vi "PH_PPMA_PowerUnit.PS Stand by.vi"(0 "i ref in":refnum<vi>, 5 "error in (no error)":errorcluster) -> (14 "i ref out":refnum<vi>, 19 "error out":errorcluster)   [LabVIEW 2014, in "PH_PPMA_PowerUnit.lvlib"]
doc: "This is the entry action of the \"Stand by\" state of the state machine."
uses:
  PH_PPMA_PowerUnit.lvlib
  PH_Devices/PH_Beckhoff_PPMA-Rods/PH_Beckhoff_PPMA-Rods.lvlib
  PH_Devices/PH_Beckhoff_PP_PU/PH_Beckhoff_PP_PU.lvlib
  PH_Basics/PH_PowerUnit_BaseClass/PH_PowerUnit_BaseClass.lvlib
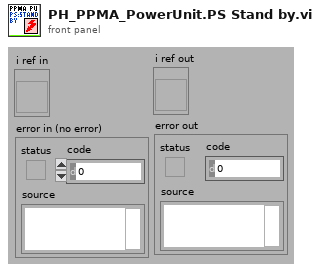
[diagram p1: front panel]
types:
  T1 = typedef "PH_PPMA_PowerUnit.lvlib/PH_PPMA_PowerUnit.i attribute.ctl" = cluster{"GUI Refs":cluster{"Rods":refnum<vi>, "Ignitron":refnum<vi>, "Rossrelais":refnum<vi>, "Set Voltage":refnum<vi>, "PSU":refnum<vi>, "EOC":refnum<vi>, "Trigger":refnum<vi>}, "Rods":T2, "PSU":T4, "Ross Relais":T5, "Ignitron":T6, "Trigger":cluster{"State Device":T3, "linked?":bool}, "Timing Settings":cluster{"Prdc Fast?":bool, "Default Value Periodic Interval":i32, "Mercury on since":dbl, "Warm up Time Mercury [s]":dbl}, "Set Voltage [V]":dbl}
  T2 = typedef "PH_PPMA_PowerUnit.lvlib/PH_PPMA_PowerUnit.Rods Attributes.ctl" = cluster{"Instancename":string, "Device Status":T3, "linked?":bool}
  T3 = typedef "PH_StatusHandler.lvlib/PH_StatusHandler.Status.ctl" = i16
  T4 = typedef "PH_PP_Common.lvlib/PH_PP_Common.PSU Attributes.ctl" = cluster{"lower limit [V]":dbl, "upper limit [V]":dbl, "Voltage set":bool, "State Device":T3, "linked?":bool}
  T5 = typedef "PH_PP_Common.lvlib/PH_PP_Common.Ross Relais Attributes.ctl" = cluster{"State Device":T3, "linked?":bool}
  T6 = typedef "PH_PP_Common.lvlib/PH_PP_Common.Ignitron Attributes.ctl" = cluster{"State Device":T3, "linked?":bool}
  T7 = typedef "PH_PowerUnit_BaseClass.lvlib/PH_PowerUnit_BaseClass.i attribute.ctl" = cluster{"Constructor finished":bool, "PU":cluster{"In use":bool, "Service ID in use":i32, "GUI Ref":refnum<vi>}, "Enabling":cluster{"State":T8, "GUI Ref":refnum<vi>}, "Timing":cluster{"Last Shot":dbl, "Time between Shots [Sec]":dbl, "Waiting Time over?":bool, "Service ID Waiting Time":i32, "GUI Ref":refnum<vi>, "Instance":cluster{"Status":T3, "linked?":bool, "GUI Ref":refnum<vi>}}, "Sequencer":cluster{"SM State":string, "GUI Ref":refnum<vi>, "linked":bool}, "Subscribed Trendmssgs":cluster{"Tagname":string, "Status":T3, "linked?":bool, "Shot Condition":T3, "GUI Ref":refnum<vi>}[], "PP PU":T9, "Default Voltage (V)":dbl, "GUI Refs":T10, "PSDB data":cluster{"Shot Voltage [V]":dbl, "State TO SM":T11, "Write 2 early":bool}, "State TO SM":T11}
  T8 = typedef "PH_SystemInformation.lvlib/PH_SystemInformationEnabling State.ctl" = i32
  T9 = typedef "PH_PP_Common.lvlib/PH_PP_Common.PUs.ctl" = enum16{"no Info", "PA-19mm-1", "PA-19mm-2", "PA-45mm-PILC", "PA-45mm-MAIN", "MA-PU-1", "MA-PU-2", "MA-PU-3", "MA-PU-4", "MA-PU-5", "MA-PU-6", "MA-FR", "MA-PILC", "PA-45mm-DP"}
  T10 = typedef "PH_PowerUnit_BaseClass.lvlib/PH_PowerUnit_BaseClass.GUI Refs.ctl" = cluster{"Delete Inst":refnum<vi>, "State TO SM":refnum<vi>, "State SM":refnum<vi>, "Fire":refnum<vi>}
  T11 = typedef "PH_PowerUnit_BaseClass.lvlib/PH_PowerUnit_BaseClass.SM States.ctl" = enum16{".", "Stand by", "Switch PU on", "Configure", "Set Default Voltage", "Set STANDBY", "Set READY", "Wait for Shot Cmd", "Open Dump Rods", "Open Ross Relais", "Close Ross Relais", "Switch PSU on", "Switch PSU off", "Charge", "Switch GD Channel on", "Close Dump Rods", "Rods-TO", "RR-TO", "PSU-TO", "Trigger-TO"}
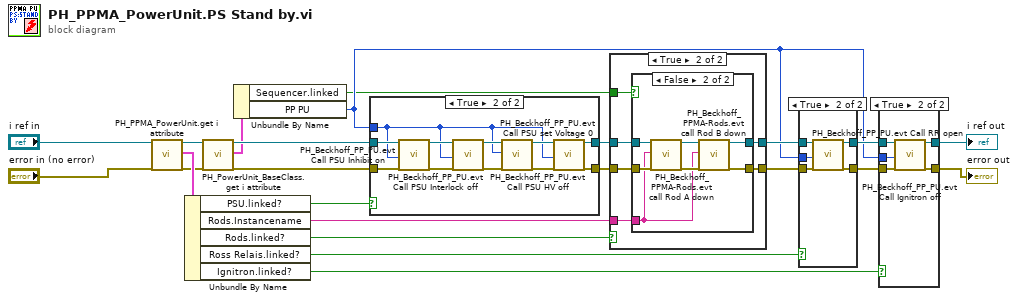
[diagram p0: block diagram]
diagram:
  n1 = call "PH_PPMA_PowerUnit.get i attribute.vi"("i ref in"="i ref in", "error in (no error)"="error in (no error)") -> ("i ref out"=w7:refnum<vi>, "i attribute"=w20:T1, "error out"=w16:errorcluster)  [unwired: 15 in]
  n2 = Unbundle By Name(w20) -> ("PSU.linked?"=w12:bool, "Rods.Instancename"=w21:string, "Rods.linked?"=w11:bool, "Ross Relais.linked?"=w10:bool, "Ignitron.linked?"=w9:bool)
  n3 = call "PH_PowerUnit_BaseClass.get i attribute.vi"("i ref in"=w7, "error in (no error)"=w16) -> ("i ref out"=w6:refnum<vi>, "i attribute"=w5:T7, "error out"=w8:errorcluster)  [unwired: 15 in]
  n4 = Unbundle By Name(w5) -> ("Sequencer.linked"=w3:bool, "PP PU"=w4:T9)
  n5 = case shown="True" w12 {
    tunnel: w6 -> [w25 w36]
    tunnel: [w25 w32] -> w13
    tunnel: w8 -> [w24 w31]
    tunnel: [w24 w27] -> w17
    tunnel: w4 -> [_ w26]
    frame False {
    }
    frame True {
      n6 = call "PH_Beckhoff_PP_PU.evt Call PSU Inhibit on.vi"("i ref in"=w36, "PU"=w26, "error in"=w31) -> ("i ref out"=w35:refnum<vi>, "error out"=w30:errorcluster)  [unwired: 15 in]
      n7 = call "PH_Beckhoff_PP_PU.evt Call PSU Interlock off.vi"("i ref in"=w35, "PU"=w26, "error in"=w30) -> ("i ref out"=w34:refnum<vi>, "error out"=w29:errorcluster)  [unwired: 15 in]
      n8 = call "PH_Beckhoff_PP_PU.evt Call PSU set Voltage 0.vi"("i ref in"=w34, "PU"=w26, "error in"=w29) -> ("i ref out"=w33:refnum<vi>, "error out"=w28:errorcluster)  [unwired: 15 in]
      n9 = call "PH_Beckhoff_PP_PU.evt Call PSU HV off.vi"("i ref in"=w33, "PU"=w26, "error in"=w28) -> ("i ref out"=w32:refnum<vi>, "error out"=w27:errorcluster)  [unwired: 15 in]
    }
  }
  n10 = case shown="True" w11 {
    tunnel: w13 -> [w38 w44]
    tunnel: [w38 w43] -> w14
    tunnel: w17 -> [w37 w42]
    tunnel: [w37 w41] -> w18
    tunnel: w21 -> [_ w40]
    tunnel: w3 -> [_ w39]
    frame False {
    }
    frame True {
      n11 = case shown="False" w39 {
        tunnel: w44 -> [w45 w53]
        tunnel: [w45 w48] -> w43
        tunnel: w42 -> [w46 w52]
        tunnel: [w46 w50] -> w41
        tunnel: w40 -> [_ w47]
        frame True {
        }
        frame False {
          n12 = call "PH_Beckhoff_PPMA-Rods.evt call Rod A down.vi"("i ref in"=w53, "Instance name"=w47, "error in"=w52) -> ("i ref out"=w49:refnum<vi>, "error out"=w51:errorcluster)  [unwired: 15 in]
          n13 = call "PH_Beckhoff_PPMA-Rods.evt call Rod B down.vi"("i ref in"=w49, "Instance name"=w47, "error in"=w51) -> ("i ref out"=w48:refnum<vi>, "error out"=w50:errorcluster)  [unwired: 15 in]
        }
      }
    }
  }
  n14 = case shown="True" w10 {
    tunnel: w14 -> [w55 w60]
    tunnel: [w55 w59] -> w15
    tunnel: w18 -> [w54 w58]
    tunnel: [w54 w57] -> w19
    tunnel: w4 -> [_ w56]
    frame False {
    }
    frame True {
      n15 = call "PH_Beckhoff_PP_PU.evt Call RR open.vi"("i ref in"=w60, "PU"=w56, "error in"=w58) -> ("i ref out"=w59:refnum<vi>, "error out"=w57:errorcluster)  [unwired: 15 in]
    }
  }
  n16 = case shown="True" w9 {
    tunnel: w15 -> [w62 w67]
    tunnel: [w62 w66] -> w23
    tunnel: w19 -> [w61 w65]
    tunnel: [w61 w64] -> w22
    tunnel: w4 -> [_ w63]
    frame False {
    }
    frame True {
      n17 = call "PH_Beckhoff_PP_PU.evt Call Ignitron off.vi"("i ref in"=w67, "PU"=w63, "error in"=w65) -> ("i ref out"=w66:refnum<vi>, "error out"=w64:errorcluster)  [unwired: 15 in]
    }
  }
  "error out" <- w22
  "i ref out" <- w23
